vi "mysql_func_escape_sql.vi"(10 "error in (no error)":errorcluster, 11 "sqlin":string) -> (2 "error out":errorcluster, 3 "escaped":string)   [LabVIEW 2014, in "FRCts20_Backend_Engine.lvlib"]
doc: "Removes any single quotes (') and thingies (`) from a sql string. There are more restricted chars, but I didn't want to waste cpu time. Only use this for custom notes,etc--any time the user can enter text that will go to the database."
uses:
  FRCts20_Backend_Engine.lvlib
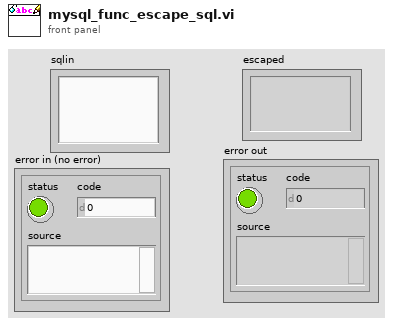
[diagram p1: front panel]
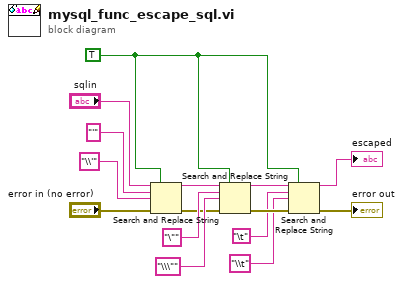
[diagram p0: block diagram]
diagram:
  w4 = TRUE ("replace all? (F)")
  n1 = Search and Replace String(replace all?=w4, input string="sqlin", search string="'", replace string="\\'" ("replace string (\"\")"), error in="error in (no error)") -> (result string=w5:string, error out=w6:errorcluster)  [unwired: 3 in, 2 out]
  n2 = Search and Replace String(replace all?=w4, input string=w5, search string="\"", replace string="\\\"" ("replace string (\"\")"), error in=w6) -> (result string=w13:string, error out=w12:errorcluster)  [unwired: 3 in, 2 out]
  n3 = Search and Replace String(replace all?=w4, input string=w13, search string="\t", replace string="\\t" ("replace string (\"\")"), error in=w12) -> (result string=→"escaped":string, error out=→"error out":errorcluster)  [unwired: 3 in, 2 out]
